vi "Send Receive.vi"   [LabVIEW 2015]
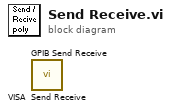
[diagram p0: block diagram]
diagram:
  n1 = call "VISA  Send Receive.vi"() -> ()  [unwired: 9 in, 3 out]
  n2 = call "GPIB Send Receive.vi"() -> ()  [unwired: 9 in, 3 out]
